vi "WF - Remove Specific Char from Signal Name.vi"(0 "wForm IN":waveform(dbl), 5 "error in (no error)":errorcluster, 7 "Characters to remove":string[](array[string]), 9 "Replace with":string=" ") -> (14 "wForm OUT":waveform(dbl), 19 "error out":errorcluster)   [LabVIEW 2020, in "GSwFormDSP.lvclass"]
uses:
  GSwFormDSP.lvclass
  functions/Attribute List.ctl
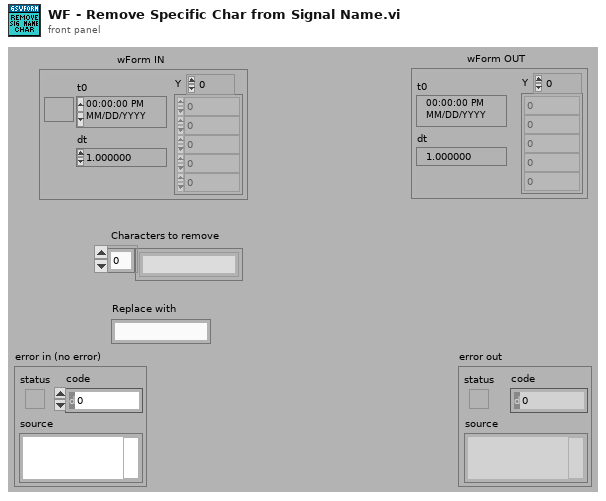
[diagram p1: front panel]
types:
  T1 = typedef "GSwFormDSP.lvclass/Attribute List.ctl" = string
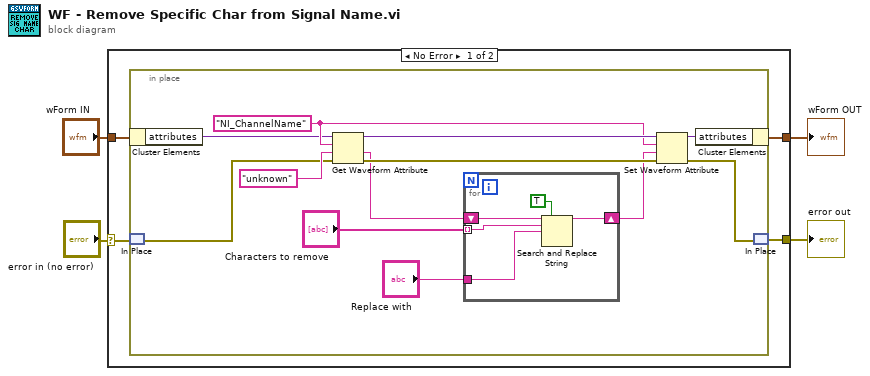
[diagram p0: block diagram]
diagram:
  n1 = case shown="No Error" "error in (no error)" {
    selector: "error in (no error)" -> [w7 w27]
    tunnel: [w5 w27] -> w3
    tunnel: [w6 w26] -> w1
    tunnel: "wForm IN" -> [w8 w26]
    frame No Error {
      n2 = in-place {
        w16 = T1 "NI_ChannelName" ("wForm Attributes")
        n3 = in-place-cluster #1(w8) -> ("attributes"=w13:variant)
        n4 = in-place-match #2(w7) -> (w14:errorcluster)
        n5 = Get Waveform Attribute(4:w14, 5:"unknown", 6:w16, 7:w13) -> (0:w15:errorcluster, 1:w12:string, 3:w17:variant)  [unwired: 1 out]
        n6 = for {
          shift-right: [w23] -> w10
          shift-left: w12 -> [w24]
          tunnel: "Characters to remove" -> [w22] mode=indexing
          tunnel: "Replace with" -> [w21]
          n7 = Search and Replace String(replace all?=TRUE ("replace all? (F)"), input string=w24, search string=w22, replace string=w21) -> (result string=w23:string)  [unwired: 4 in, 3 out]
        }
        n8 = Set Waveform Attribute(4:w15, 5:w10, 6:w16, 7:w17) -> (0:w19:errorcluster, 3:w20:variant)  [unwired: 1 out]
        n9 = in-place-cluster #1("attributes"=w20) -> (w6:waveform(dbl))
        n10 = in-place-match #2(w19) -> (w5:errorcluster)
      }
    }
    frame Error {
    }
  }
  "error out" <- w3
  "wForm OUT" <- w1
